vi "count.vi"(8 "error in (no error)":errorcluster, 11 "VGS_ComponentInfo in":refnum<class "VGS_ComponentInfo.lvclass">) -> (0 "error out":errorcluster, 2 "count":i32, 3 "VGS_ComponentInfo out":refnum<class "VGS_ComponentInfo.lvclass">)   [LabVIEW 2022 SP3, in "LV_VGS.lvlib" / "VGS_ComponentInfo.lvclass"]
uses:
  VGS_ComponentInfo.lvclass
  VGS_ComponentInfo.lvclass/VGS_ComponentInfo.ctl
  C:/Users/Andrey/Desktop/hajo/LV_VGS/vgs_project.dll
  vgs_project.dll
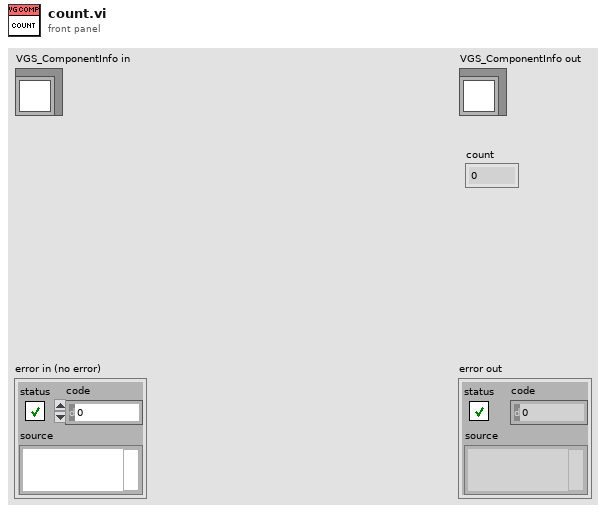
[diagram p1: front panel]
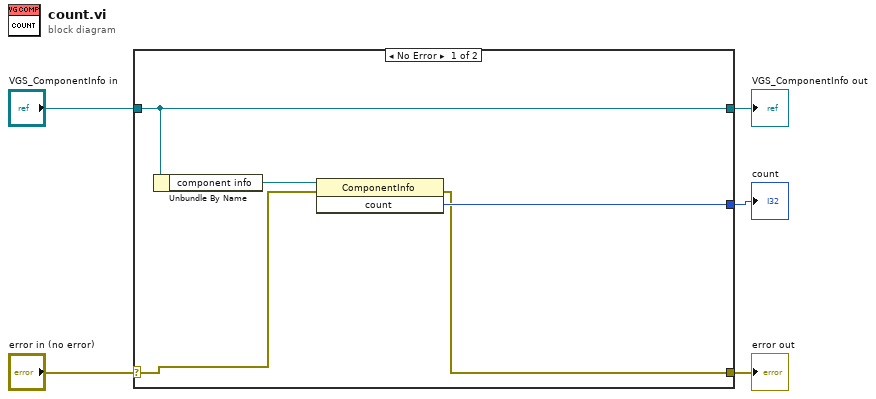
[diagram p0: block diagram]
diagram:
  n1 = case shown="No Error" "error in (no error)" {
    selector: "error in (no error)" -> [w7 w12]
    tunnel: [w6 w12] -> w4
    tunnel: [w10 w11] -> w2
    tunnel: "VGS_ComponentInfo in" -> [w10 w11]
    tunnel: [w8 _] -> w1
    frame No Error {
      n2 = Unbundle By Name(w10) -> ("component info"=w9:refnum<k24>)
      n3 = invoke class="ComponentInfo" method="count"(reference=w9, error in=w7) -> (error out=w6:errorcluster, "count"=w8:i32)  [unwired: 1 in, 1 out]
    }
    frame Error {
    }
  }
  "error out" <- w4
  "VGS_ComponentInfo out" <- w2
  "count" <- w1
